vi "10-Tap 8-bit Camera without DRAM (FPGA-SIM)RandomSimDataNoAccumulation.vi"() -> ()   [LabVIEW 2013]
doc: "This is the FPGA VI for the 10-Tap 8-Bit Camera with DRAM example. This example demonstrates how to acquire images from a 10-tap, 8-bit, extended configuration, Camera Link camera and transfer the images to the host. This example supports area scan and line scan cameras for both continuous and finite acquisitions.\n\nThis example also demonstrates the use of DRAM as a frame buffer for very high speed acquisitions. Data packing and flow-control are also employed to maximize use of the available DRAM and FIFOs in terms of both memory space and performance.\n\nAdditionally, the example demonstrates the serial server, which allows third-party camera configuration utilities to communicate with the camera using the Camera Link serial interface while this VI is running."
uses:
  <vilib>/rvi/DataTransferAndStorage/Container/XNode/niFpgaContainer.xnode
  <vilib>/Platform/TimedLoop/XDataNode/XDataNode.xnode
  <vilib>/Platform/TimedLoop/XDataNode/timing_clust.ctl
  <vilib>/Platform/TimedLoop/XDataNode/XDNodeRunTimeDep.lvlib
  <vilib>/Platform/TimedLoop/XDataNode/wakeup.ctl
  <vilib>/Platform/TimedLoop/XDataNode/nitl_modes.ctl
  <vilib>/rvi/FIFO/Fifo_Resource/nirvififoEmulationRead.vi
  <vilib>/rvi/FIFO/Fifo_Resource/nirvififoEmulationWrite.vi
  FPGA/Globals/Accumulated Sector Intensity.vi
  FPGA/Globals/Pixel Location Global.vi
  FPGA/Globals/Wing Square Wave Frequency Global.vi
  FPGA/Globals/Sector Parameter Global.vi
  <vilib>/rvi/FIFO/Fifo_Resource/nirvififoEmulationGetNumberOfElementsToWrite.vi
  <vilib>/rvi/FIFO/Fifo_Resource/nirvififoEmulationGetNumberOfElementsToRead.vi
  <vilib>/rvi/interface/RandomDataEmulation/nirviRandomDataFpgaReadWriteTemplate.vi
  Common/CL Signal Mapping.ctl
  Common/CL Configuration.ctl
  FPGA/Sector/Accumulate/Sector Parameter Cluster.ctl
panel:
  in  "Sim Data":u64=44
  out "Number of Elements to Write Sector Grouping FIFO":u32
  out "Accumulate Ticks":u32
  out "Analysis Ticks":u32
  out "Target Sim TO":bool
  out "Cam Data Timeout":bool
  out "Sector FIFO Timeout":bool
  out "Host DMA Timeout":bool
  out "Number of Elements to Read Cam Data":u32
  out "Number of Elements to Write Host DMA":u32
  in  "Words per image":u32=1000
  in  "Y Resolution":u16=1000
  in  "X Resolution":u16=1000
  in  "[Average BG Intensity]":u8[](array[numeric])=[0, 0, 0, 0, 0, 0, 0, 0, 0, 0, 0, 0, 0, 0, 0, 0, 0, 0, 0, 0, 0, 0, 0, 0, 0, 0, 0, 0, 0, 0, 0, 0]
  in  "Sector Threshold":u8
  in  "# of Frames to Average":u8=1
  in  "Sector Parameters Right":T1={"Start Angle"=0.0, "End Angle"=0.4708251953125, "Inner Radius"=309, "Outter Radius"=405, "Hinge X"=685, "Hinge Y"=527, "NumWingSectors"=8}
  in  "Sector Parameters Left":T1={"Start Angle"=0.65740966796875, "End Angle"=0.99468994140625, "Inner Radius"=309, "Outter Radius"=405, "Hinge X"=464, "Hinge Y"=534, "NumWingSectors"=8}
  in  "CL Config.Configuration":T2=enum."Full"
  in  "CL Config.Signal Mapping":T3=enum."Basler 10-tap"
  in  "CL Config.Line Scan":bool
  in  "CL Config.DVAL Active High":bool=TRUE
  in  "CL Config.LVAL Active High":bool=TRUE
  in  "CL Config.FVAL Active High":bool=TRUE
  in  "CL Config.Spare Active High":bool=TRUE
  in  "Acq Control.Line Scan Height":u32
  in  "Acq Control.Frames To Acq":u32
  in  "Acq Control.Acquire":bool
  in  "Acq Control.Cancel Acq":bool
  in  "Acq Control.Ignore DVAL":bool
  in  "Acq Control.Initialize":bool
  out "Acq Status.Acq In Progress":bool
  out "Acq Status.Clocks Per Line":u32
  out "Acq Status.Frames Acq'd":u32
  out "Acq Status.Lines Per Frame":u32
  out "Acq Status.DMA Write Timeout":bool
  out "Acq Status.Initialized":bool
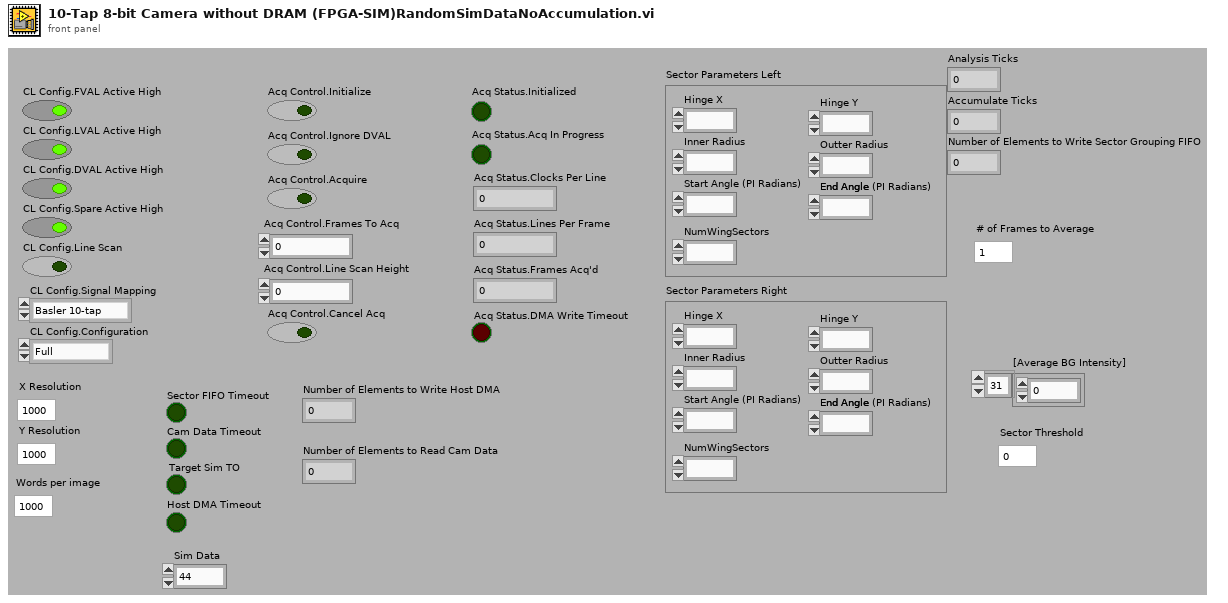
[diagram p1: front panel]
types:
  T1 = typedef "Sector Parameter Cluster.ctl" = cluster{"Start Angle":fxp<+/-,17,2>, "End Angle":fxp<+,17,3>, "Inner Radius":u16, "Outter Radius":u16, "Hinge X":u16, "Hinge Y":u16, "NumWingSectors":u8}
  T2 = typedef "CL Configuration.ctl" = enum8{"Base", "Medium", "Full"}
  T3 = typedef "CL Signal Mapping.ctl" = enum8{"Standard", "Basler 10-tap", "Vosskühler 10-tap"}
  T4 = typedef "XDNodeRunTimeDep.lvlib/timing_clust.ctl" = cluster{"Expected End [f-1]":u64, "Actual End [f-1]":u64, "Finished Late? [f-1]":bool, "Expected End [i-1]":u64, "Actual End [i-1]":u64, "Finished Late? [i-1]":bool, "Expected Start [i]":u64, "Actual Start [i]":u64, "Expected Start [f]":u64, "Actual Start [f]":u64, "Source Name":string, "Structure Name":string, "Period":i64, "Deadline":i64, "Offset":i64, "Start":i64, "Priority":i32, "Timeout":i32, "Mode":T5, "Wakeup Reason":T6, "Error":errorcluster, "Source Type":string, "Secondary Source Type":string, "Global End Time":u64, "Global Start Time":u64, "Frame Duration":u64, "Iteration Duration":u64, "Assigned CPU":i32, "I/O Scan Engine Mode":u32}
  T5 = typedef "XDNodeRunTimeDep.lvlib/nitl_modes.ctl" = enum32{"No Change", "Process missed periods, maintain original phase", "Discard missed periods, maintain original phase", "Process missed periods, ignore original phase", "Discard missed periods, ignore original phase"}
  T6 = typedef "XDNodeRunTimeDep.lvlib/wakeup.ctl" = enum32{"Normal", "Aborted", "Asynchronous wakeup", "Timing source error", "Timed loop error", "Timeout"}
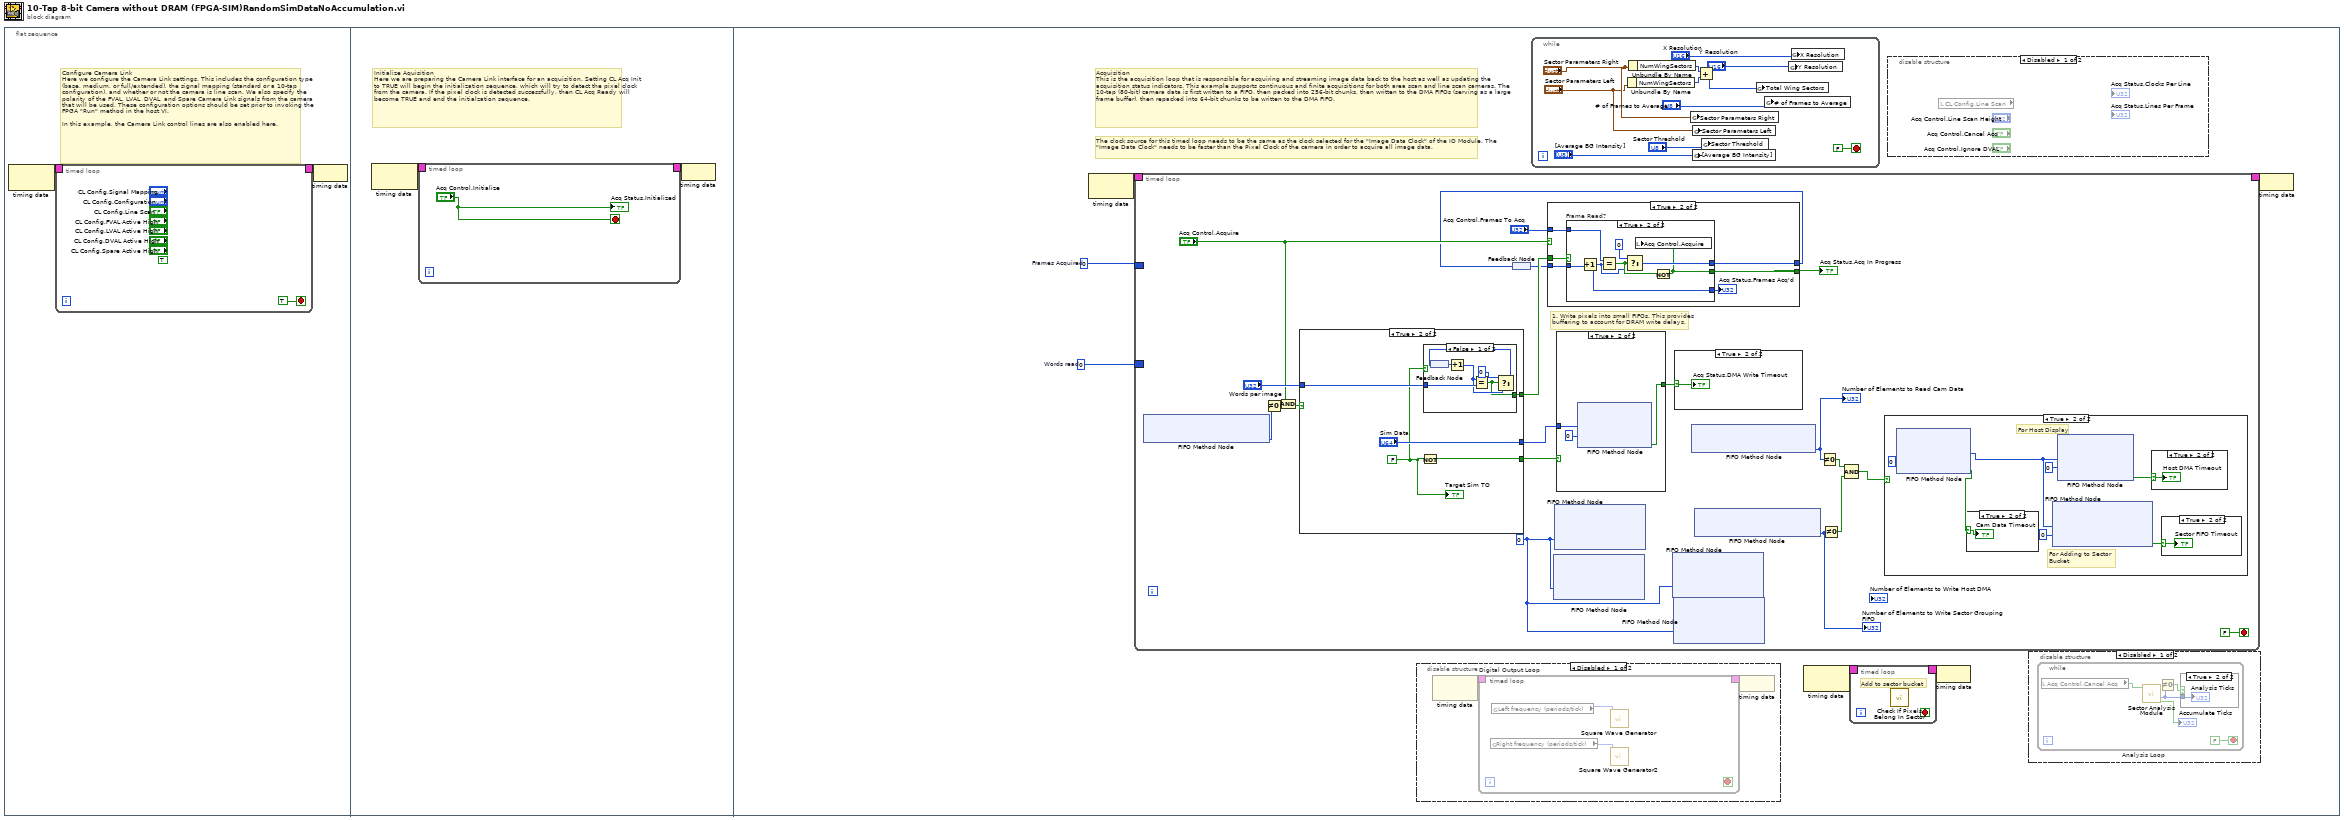
[diagram p0: block diagram]
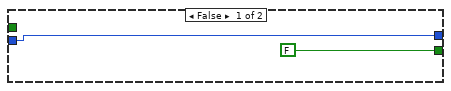
[diagram p7: hidden frame]
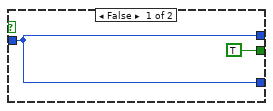
[diagram p8: hidden frame]
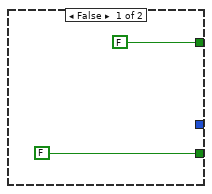
[diagram p9: hidden frame]
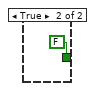
[diagram p10: hidden frame]
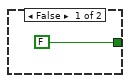
[diagram p15: hidden frame]
diagram:
  n1 = flat-sequence {
    frame #0 {
      # "Configure Camera Link\nHere we configure the Camera Link settings. This includes the configuration type (base, medium, or full/extended), the signal mapping (standard or a 10-tap configuration), and whether or not the camera is line scan. We also specify the polarity of the FVAL, LVAL, DVAL, and Spare Camera Link signals from the camera that will be used. These configuration options should be set prior to invoking the FPGA \"Run\" method in the host VI.\n\nIn this example, the Camera Link control lines are also enabled here."
      n2 = node-c288() -> (w2:T4)  [unwired: 1 in]
      n3 = timed-loop {
        timing: w2 -> [_]
        timing-out: [_] -> w1
        stop <- TRUE stop-if-true
        (unwired) TRUE ("IO Module\\CL Control Enable")
      }
      n4 = node-c288(w1) -> ()
    }
    frame #1 {
      # "Initialize Aquisition\nHere we are preparing the Camera Link interface for an acquisition. Setting CL Acq Init to TRUE will begin the initialization sequence, which will try to detect the pixel clock from the camera. If the pixel clock is detected successfully, then CL Acq Ready will become TRUE and end the initialzation sequence."
      n5 = node-c288() -> (w9:T4)  [unwired: 1 out]
      n6 = timed-loop {
        timing: w9 -> [_]
        timing-out: [_] -> w8
        stop <- "Acq Control.Initialize" stop-if-true
        "Acq Status.Initialized" <- "Acq Control.Initialize"
      }
      n7 = node-c288(w8) -> ()
    }
    frame #2 {
      w17 = u32 0  # Frames Acquired
      w18 = u32 0  # Words read
      # "The clock source for this timed loop needs to be the same as the clock selected for the \"Image Data Clock\" of the IO Module. The \"Image Data Clock\" needs to be faster than the Pixel Clock of the camera in order to acquire all image data."
      # "Acquisition\nThis is the acquisition loop that is responsible for acquiring and streaming image data back to the host as well as updating the acquisition status indicators. This example supports continuous and finite acquisitions for both area scan and line scan cameras. The 10-tap (80-bit) camera data is first written to a FIFO, then packed into 256-bit chunks, then written to the DMA FIFOs (serving as a large frame buffer), then repacked into 64-bit chunks to be written to the DMA FIFO."
      n8 = node-c288() -> (w20:T4)  [unwired: 1 in]
      n9 = timed-loop {
        timing: w20 -> [_]
        timing-out: [_] -> w19
        border: w18 -> [_]
        border: w17 -> [_]
        stop <- FALSE stop-if-true
        w44 = 0 ("Timeout")
        # "1. Write pixels into small FIFOs. This provides\nbuffering to account for DRAM write delays."
        n10 = xnode ("FIFO Method Node")() -> ("Number of Elements to Write"=w54:u32)  [unwired: 1 in, 1 out]
        n11 = Not Equal To 0?(x=w54) -> (x != 0?=w53:bool)
        n12 = Compound Arithmetic op=AND("Acq Control.Acquire", w53) -> (w60:bool)
        n13 = case shown="True" w60 {
          tunnel: [_ "Sim Data"] -> w64
          tunnel: [FALSE w87] -> w62
          tunnel: "Words per image" -> [_ w89]
          tunnel: [FALSE w88] -> w50
          frame False {
          }
          frame True {
            w85 = FALSE ("x")
            n14 = Not(x=w85) -> (.not. x?=w87:bool)
            n15 = case shown="False" w85 {
              tunnel: w89 -> [w95 _]
              tunnel: [w90 FALSE] -> w88
              frame False {
                n16 = feedback #1() -> (w94:u32)
                n17 = Increment(x=w94) -> (x+1=w91:u32)
                n18 = Equal?(x=w91, y=w95) -> (x = y?=w90:bool)
                n19 = Select(t=u32 0 ("Acq Status.Frames Acq'd"), s=w90, f=w91) -> (s? t:f=w92:u32)
                n20 = feedback-in #1(w92) -> ()
              }
              frame True {
              }
            }
            "Target Sim TO" <- w85
          }
        }
        n21 = feedback #2() -> (w49:u32)
        n22 = case shown="True" "Acq Control.Acquire" {
          tunnel: w50 -> [_ w73]
          tunnel: w49 -> [w67 w72]
          tunnel: "Acq Control.Frames To Acq" -> [_ w71]
          tunnel: [w67 w70] -> w47
          tunnel: [FALSE w69] -> w46
          frame False {
          }
          frame True {
            n23 = case "Frame Read?" shown="True" w73 {
              tunnel: w72 -> [w74 w82]
              tunnel: w71 -> [_ w81]
              tunnel: [w74 w79] -> w70
              tunnel: [TRUE w77] -> w69
              tunnel: [w74 w76] -> w68
              frame False {
              }
              frame True {
                n24 = Increment(x=w82) -> (x+1=w76:u32)
                n25 = Equal?(x=w81, y=w76) -> (x = y?=w78:bool)
                n26 = Select(t=u32 0 ("Frames Acquired"), s=w78, f=w76) -> (s? t:f=w79:u32)
                n27 = Not(x=w78) -> (.not. x?=w77:bool)
                n28 = local write "Acq Control.Acquire"(w77) -> ()
              }
            }
            "Acq Status.Frames Acq'd" <- w68
          }
        }
        "Acq Status.Acq In Progress" <- w46
        n29 = feedback-in #2(w47) -> ()
        n30 = xnode ("FIFO Method Node")("Timeout"=w44) -> ()  [unwired: 1 in, 3 out]
        n31 = xnode ("FIFO Method Node")("Timeout"=w44) -> ()  [unwired: 1 in, 3 out]
        n32 = case shown="True" w62 {
          tunnel: [FALSE ("Timed Out?") w109] -> w45
          tunnel: w64 -> [_ w110]
          frame False {
          }
          frame True {
            n33 = xnode ("FIFO Method Node")("Element"=w110, "Timeout"=0) -> ("Timed Out?"=w109:bool)  [unwired: 1 in, 1 out]
          }
        }
        n34 = xnode ("FIFO Method Node")("Timeout"=w44) -> ()  [unwired: 1 in, 3 out]
        n35 = xnode ("FIFO Method Node")("Timeout"=w44) -> ()  [unwired: 1 in, 3 out]
        n36 = case shown="True" w45 {
          selector: w45 -> [_ w65]
          frame False {
          }
          frame True {
            "Acq Status.DMA Write Timeout" <- w65
          }
        }
        n37 = xnode ("FIFO Method Node")() -> ("Number of Elements to Read"=w56:u32)  [unwired: 1 in, 1 out]
        "Number of Elements to Read Cam Data" <- w56
        n38 = xnode ("FIFO Method Node")() -> ("Number of Elements to Write"=w58:u32)  [unwired: 1 in, 1 out]
        "Number of Elements to Write Sector Grouping FIFO" <- w58
        n39 = Not Equal To 0?(x=w56) -> (x != 0?=w55:bool)
        n40 = Not Equal To 0?(x=w58) -> (x != 0?=w57:bool)
        n41 = Compound Arithmetic op=AND(w55, w57) -> (w61:bool)  [unwired: 1 in]
        n42 = case shown="True" w61 {
          frame False {
          }
          frame True {
            # "For Adding to Sector \nBucket"
            # "For Host Display"
            n43 = xnode ("FIFO Method Node")("Timeout"=0) -> ("Element"=w101:u64, "Timed Out?"=w97:bool)  [unwired: 1 in, 1 out]
            n44 = case shown="True" w97 {
              selector: w97 -> [_ w104]
              frame False {
              }
              frame True {
                "Cam Data Timeout" <- w104
              }
            }
            n45 = xnode ("FIFO Method Node")("Element"=w101, "Timeout"=0) -> ("Timed Out?"=w99:bool)  [unwired: 1 in, 1 out]
            n46 = xnode ("FIFO Method Node")("Element"=w101, "Timeout"=0) -> ("Timed Out?"=w98:bool)  [unwired: 1 in, 1 out]
            n47 = case shown="True" w98 {
              selector: w98 -> [_ w105]
              frame False {
              }
              frame True {
                "Host DMA Timeout" <- w105
              }
            }
            n48 = case shown="True" w99 {
              selector: w99 -> [_ w106]
              frame False {
              }
              frame True {
                "Sector FIFO Timeout" <- w106
              }
            }
          }
        }
      }
      n49 = disable-structure shown="Disabled" {
        frame Disabled {
          n50 = node-c288() -> (w37:T4)  [unwired: 1 in]
          n51 = timed-loop "Digital Output Loop" {
            timing: w37 -> [_]
            timing-out: [_] -> w36
            stop <- _ stop-if-true
            n52 = global read "Wing Square Wave Frequency Global.vi" "Right frequency (periods/tick)"() -> (w38:fxp<+,32,0>)
            n53 = global read "Wing Square Wave Frequency Global.vi" "Left frequency (periods/tick)"() -> (w39:fxp<+,32,0>)
            n54 = call "Square Wave Generator"("frequency (periods/tick)"=w39) -> ()  [unwired: 14 in, 1 out]
            n55 = call "Square Wave Generator2"("frequency (periods/tick)"=w38) -> ()  [unwired: 14 in, 1 out]
          }
          n56 = node-c288(w36) -> ()
        }
        frame Enabled {
        }
      }
      n57 = while {
        stop <- FALSE stop-if-true
        n58 = Unbundle By Name("Sector Parameters Left") -> ("NumWingSectors"=w123:u8)
        n59 = Unbundle By Name("Sector Parameters Right") -> ("NumWingSectors"=w124:u8)
        n60 = global write "Sector Parameter Global.vi" "Sector Parameters Right"("Sector Parameters Right") -> ()
        n61 = global write "Sector Parameter Global.vi" "Sector Parameters Left"("Sector Parameters Left") -> ()
        n62 = global write "Sector Parameter Global.vi" "[Average BG Intensity]"("[Average BG Intensity]") -> ()
        n63 = Add(x=w124, y=w123) -> (x+y=w122:u8)
        n64 = global write "Sector Parameter Global.vi" "Sector Threshold"("Sector Threshold") -> ()
        n65 = global write "Accumulated Sector Intensity.vi" "Total Wing Sectors"(w122) -> ()
        n66 = global write "Pixel Location Global.vi" "# of Frames to Average"("# of Frames to Average") -> ()
        n67 = global write "Pixel Location Global.vi" "Y Resolution"("Y Resolution") -> ()
        n68 = global write "Pixel Location Global.vi" "X Resolution"("X Resolution") -> ()
      }
      n69 = node-c288() -> (w16:T4)  [unwired: 1 in]
      n70 = timed-loop {
        timing: w16 -> [_]
        timing-out: [_] -> w15
        stop <- _ stop-if-true
        # "Add to sector bucket"
        n71 = call "Check If Pixels Belong In Sector.vi"() -> ()  [unwired: 11 in, 1 out]
      }
      n72 = disable-structure shown="Disabled" {
        frame Disabled {
          n73 = local read "CL Config.Line Scan"() -> (w33:bool)
        }
        frame Enabled {
        }
      }
      n74 = node-c288(w15) -> ()
      n75 = disable-structure shown="Disabled" {
        frame Disabled {
          n76 = while "Analysis Loop" {
            stop <- FALSE stop-if-true
            n77 = local read "Acq Control.Cancel Acq"() -> (w24:bool)
            n78 = call "Sector Analysis Module.vi"("Canceled?"=w24) -> ("New Data? Out"=→"Accumulate Ticks":bool, "Analysis Ticks"=w22:u32)  [unwired: 6 in, 3 out]
            n79 = Not Equal To 0?(x=w22) -> (x != 0?=w21:bool)
            n80 = case shown="True" w21 {
              tunnel: w22 -> [_ w26]
              frame False {
              }
              frame True {
                "Analysis Ticks" <- w26
              }
            }
          }
        }
        frame Enabled {
        }
      }
      n81 = node-c288(w19) -> ()
    }
  }
